vi "Init Guardian List.vi"(8 "error in (no error)":errorcluster, 11 "Guardian in":refnum<class "Guardian.lvclass">) -> (0 "error out":errorcluster, 3 "Guardian out":refnum<class "Guardian.lvclass">)   [LabVIEW 2026, in "TALOS.lvlib" / "Guardian.lvlib" / "Guardian.lvclass"]
doc: "This VI initialise the Guardian List (for now, it only populates the names)."
uses:
  Guardian.lvclass
  Guardian.lvclass/Guardian.ctl
  Classes/Guardian List/Guardian Properties.ctl
  Ancestor/Ancestor/Ancestor.lvclass/Ancestor.ctl
  Support VIs/Circus Config Param - Core.vi
  Support VIs/Generate Error.vi
  Support VIs/Circus Root Path.vi
  Support VIs/TALOS Config Param.vi
  FGV/Error Memory/Get Error Description.vi
  Support VIs/Get PC name.vi
  Ancestor/Ancestor/Read ID.vi
  Support VIs/Get Class Name.vi
  <vilib>/Utility/error.llb/Clear Errors.vi
  FGV/Error Memory/Error Memory Core.vi
  <vilib>/AdvancedString/Delimited String to 1D String Array.vi
  <vilib>/AdvancedString/Delimited String to 1D String Array (string).vi
  FGV/Error Memory/Error Crt Lvl checker.vi
  FGV/Error Memory/Error Memory Core.vi/40c8088d-b597-4017-91af-faa98e00292e.vi
  FGV/Error Memory/Error Memory Core.vi/d4a3ab98-063c-4e44-b43d-fbdcfe6c2be2.vi
  Support VIs/Global Constants.vi
  Support VIs/Global Memory.vi
  <vilib>/Utility/LVClass/Get LV Class Name.vi
  Support VIs/Is in Packed Library.vi
  Support VIs/TALOS Root path.vi
  Support VIs/Read CSV worksheet.vi
  <vilib>/Utility/error.llb/General Error Handler.vi
  <vilib>/Utility/config.llb/Open Config Data.vi
  <vilib>/Utility/config.llb/Get Section Names.vi
  <vilib>/Utility/config.llb/Get Key Names.vi
  <vilib>/Utility/config.llb/Read Key.vi
  <vilib>/Utility/config.llb/Read Key (String).vi
  <vilib>/Utility/config.llb/Close Config Data.vi
  Extract list from Project INI file entry.vi
  Ancestor/Ancestor/Ancestor.lvclass
  <vilib>/Comparison/Equal/Equal Functor/Equal Functor.lvclass
  Classes/Guardian List/Guardian List.lvclass
  TALOS.lvlib
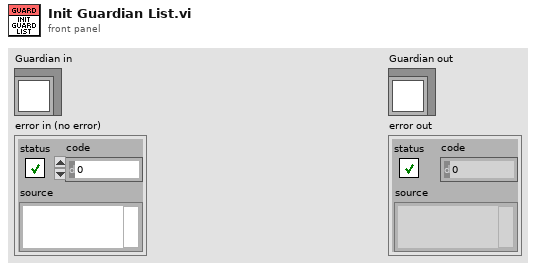
[diagram p1: front panel]
types:
  T1 = typedef "TALOS.lvlib/Classes.lvlib/Guardian List.lvclass/Guardian Properties.ctl" = cluster{"Alive":bool, "Last Seen":timestamp, "IP":string, "TCP Writer associated ID":string, "uS List received":bool, "Abort":bool, "Bearer":bool, "TCP Listener associated ID":string}
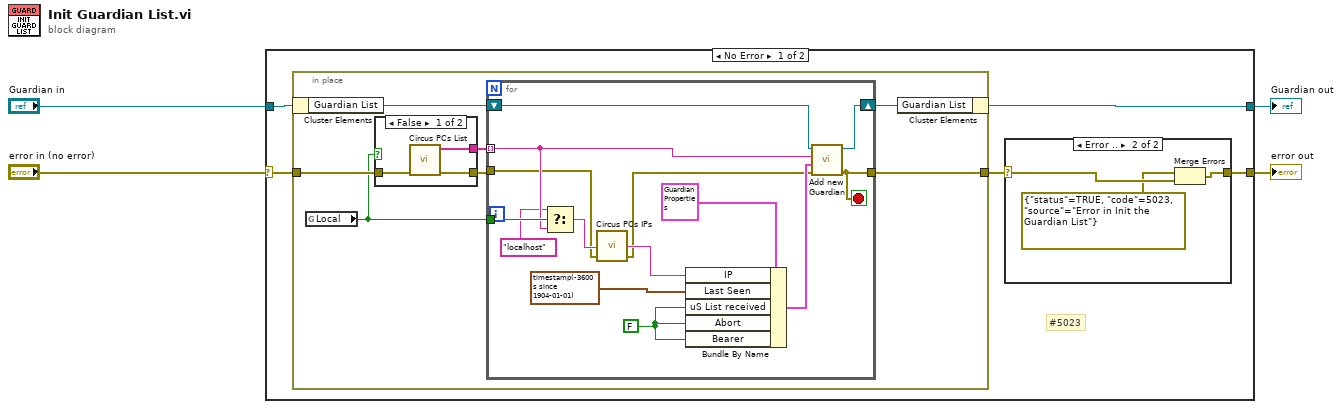
[diagram p0: block diagram]
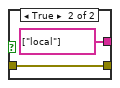
[diagram p2: hidden frame]
diagram:
  n1 = case shown="No Error" "error in (no error)" {
    selector: "error in (no error)" -> [w9 w40]
    tunnel: [w5 w40] -> w3
    tunnel: "Guardian in" -> [w6 w41]
    tunnel: [w7 w41] -> w1
    frame No Error {
      # "#5023"
      n2 = in-place {
        in-place-border: w9 -> [w11]
        in-place-border: [w16] -> w8
        n3 = in-place-cluster #1(w6) -> ("Guardian List"=w14:refnum<class "Guardian List.lvclass">)
        n4 = global read "Global Constants.vi" "Local"() -> (w10:bool)
        n5 = case shown="False" w10 {
          tunnel: [w19 w21] -> w15
          tunnel: [w18 string[] ["local"] ("PC List out")] -> w12
          tunnel: w11 -> [w17 w21]
          frame False {
            n6 = call "Circus PCs List.vi"("error in (no error)"=w17) -> ("error out"=w19:errorcluster, "PC List out"=w18:string[])  [unwired: 9 in]
          }
          frame True {
          }
        }
        n7 = for {
          shift-right: [w34] -> w13
          shift-left: w14 -> [w35]
          tunnel: w12 -> [w30] mode=indexing
          tunnel: w10 -> [w31]
          tunnel: w15 -> [w25]
          tunnel: [w23] -> w16
          stop <- w23 stop-if-true
          w22 = FALSE ("uS List received")
          n8 = Select(t="localhost", s=w31, f=w30) -> (s? t:f=w28:string)
          n9 = call "Circus PCs IPs.vi"("error in (no error)"=w25, "ID"=w28) -> ("error out"=w24:errorcluster, "IP"=w27:string)  [unwired: 2 in]
          n10 = Bundle By Name(cluster=T1 {"Alive"=FALSE, "Last Seen"=timestamp(0 s since 1904-01-01), "IP"="", "TCP Writer associated ID"="", "uS List received"=FALSE, "Abort"=FALSE, "Bearer"=FALSE, "TCP Listener associated ID"=""} ("Guardian Properties"), "IP"=w27, "Last Seen"=timestamp(-3600 s since 1904-01-01), "uS List received"=w22, "Abort"=w22, "Bearer"=w22) -> (w32:T1)
          n11 = call-dynamic "Add new Guardian.vi"("error in (no error)"=w24, "Guardian Properties"=w32, "ID"=w30, "Guardian List in"=w35) -> ("error out"=w23:errorcluster, "Guardian List out"=w34:refnum<class "Guardian List.lvclass">)  [unwired: 6 in]
        }
        n12 = in-place-cluster #1("Guardian List"=w13) -> (w7:refnum<class "Guardian.lvclass">)
      }
      n13 = case shown="Error .." w8 {
        selector: w8 -> [w36 w39]
        tunnel: [w36 w38] -> w5
        frame No Error {
        }
        frame Error {
          n14 = Merge Errors(errorcluster {"status"=TRUE, "code"=5023, "source"="Error in Init the Guardian List"} ("error in"), w39) -> (w38:errorcluster)
        }
      }
    }
    frame Error {
    }
  }
  "Guardian out" <- w1
  "error out" <- w3
